vi "Config_interface.vi"() -> ()   [LabVIEW 2015]
uses:
  <vilib>/Utility/config.llb/NI_LVConfig.lvlib
  <vilib>/Utility/config.llb/Write Key (Double).vi
  <vilib>/Utility/config.llb/Write Key (String).vi
  <vilib>/Utility/config.llb/Write Key (U32).vi
  <vilib>/Utility/config.llb/Write Key (Boolean).vi
  <vilib>/LabVIEW Targets/FPGA/cRIO/shared/nicrio_ModuleControls/nicrio_cRIO-9233_DataRatesRing.ctl
panel:
  in  "Ruta en la que se quiere guardar el archivo parametros.cfg":path=path "Parametros.cfg"
  in  "Días entre TEST":i16(slide) scale=0.0..50.0
  in  "Horario":cluster{sgl, sgl, sgl}(slide)={61389.473, 53948.324, 46173.875} scale=0.0..86400.0 scale format="%<%H:%M>t"
  in  "Tab Control":T1(tab)=enum."Parámetros"
  in  "Frecuencia de muestreo (Hz)":dbl=50000.0
  in  "Escaneos de la FIFO por canal":u32=1000
  in  "Tiempo extra al detector de paso (s)":dbl=1.0
  in  "Filtro digital (ms)":u16=13
  in  "dt RMS":dbl=500.0
  in  "Data Rate":T2=2 items=["50.000 kS/s (NI 9233)"=2, "33.333 kS/s (NI 9233)"=3, "25.000 kS/s (NI 9233)"=34, "16.667 kS/s (NI 9233)"=35, "12.500 kS/s (NI 9233)"=36, "10.000 kS/s (NI 9233)"=37, "  8.333 kS/s (NI 9233)"=38, "  7.143 kS/s (NI 9233)"=39, "  6.250 kS/s (NI 9233)"=40, "  5.556 kS/s (NI 9233)"=41, "  5.000 kS/s (NI 9233)"=42, "  4.545 kS/s (NI 9233)"=43, "  4.167 kS/s (NI 9233)"=44, "  3.846 kS/s (NI 9233)"=45, "  3.571 kS/s (NI 9233)"=46, "  3.333 kS/s (NI 9233)"=47, "  3.125 kS/s (NI 9233)"=48, "  2.941 kS/s (NI 9233)"=49, "  2.778 kS/s (NI 9233)"=50, "  2.632 kS/s (NI 9233)"=51, "  2.500 kS/s (NI 9233)"=52, "  2.381 kS/s (NI 9233)"=53, "  2.273 kS/s (NI 9233)"=54, "  2.174 kS/s (NI 9233)"=55, "  2.083 kS/s (NI 9233)"=56, "  2.000 kS/s (NI 9233)"=57]
  in  "Puerto de conexión RFID":u16=2189
  in  "IP de RFID":string="192.168.100.2"
  in  "Hora de descarga":string="HH:MM"
  in  "Periodo descarga\n (Días)":u16=3
  in  "Descarga automática 2":bool
  in  "Hora de descarga":string="HH:MM"
  in  "Descarga automática":bool
  in  "Password FTP":string="crioftp"
  in  "Username FTP":string="crioftp"
  in  "Puerto FTP":u16=2121
  in  "IP del servidor FTP":string="80.39.98.109"
  in  "Puerto TCP/IP":u16=2122
  in  "IP del servidor FTP 2":string="80.39.98.109"
  in  "Username FTP 2":string="crioftp"
  in  "Password FTP 2":string="crioftp"
  in  "Puerto FTP 2":u16=2121
  in  "Periodo  de borrado de\narchivos (Días)":u16=5
  out "error out":errorcluster
  out "Horario TEST":string
  out "Horario inicio":string
  out "Horario final":string
  # "Funciona?"
  # "Inductivo"
  # "A4"
  # "A3"
  # "A1"
  # "A2"
  # "Inicio"
  # "Final"
  # "TEST"
  # "Dcha"
  # "Izda"
  # "Última detección de unidad"
  # "Error!!"
  # "Estado de la memoria"
  # "Parámetros de muestreo"
  # "Parámetros de adquisición"
  # "Parámetros de RFID"
  # "Cambio Fecha y Hora"
  # "Descarga de planos y TEST"
  # "NO"
  # "SI"
  # "Descarga archivos binarios de adquisición"
  # "NO"
  # "SI"
  # "Cargar datos de configuración"
  # "Errores!!"
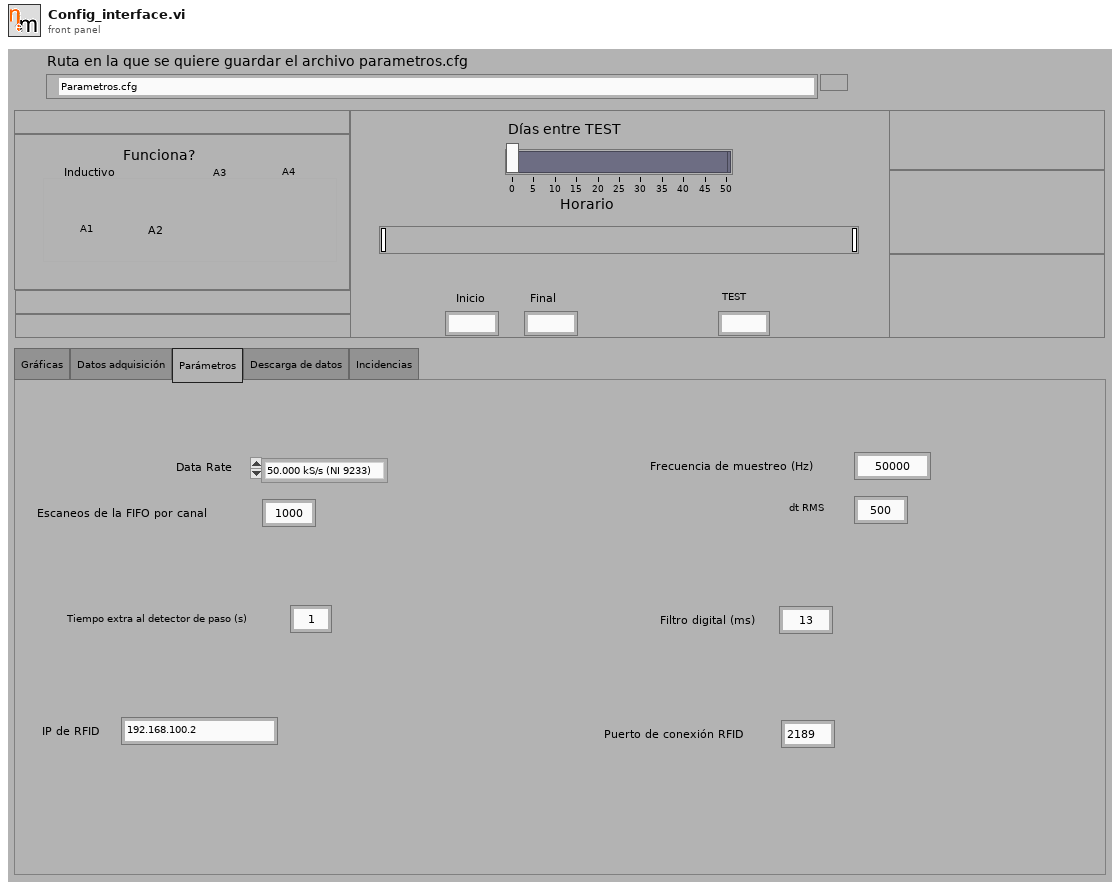
[diagram p1: front panel]
types:
  T1 = enum32{"Gráficas", "Datos adquisición", "Parámetros", "Descarga de datos", "Incidencias"}
  T2 = typedef "nicrio_cRIO-9233_DataRatesRing.ctl" = u8
  T3 = typedef "NI_LVConfig.lvlib/Config Data RefNum.ctl" = refnum<k1>
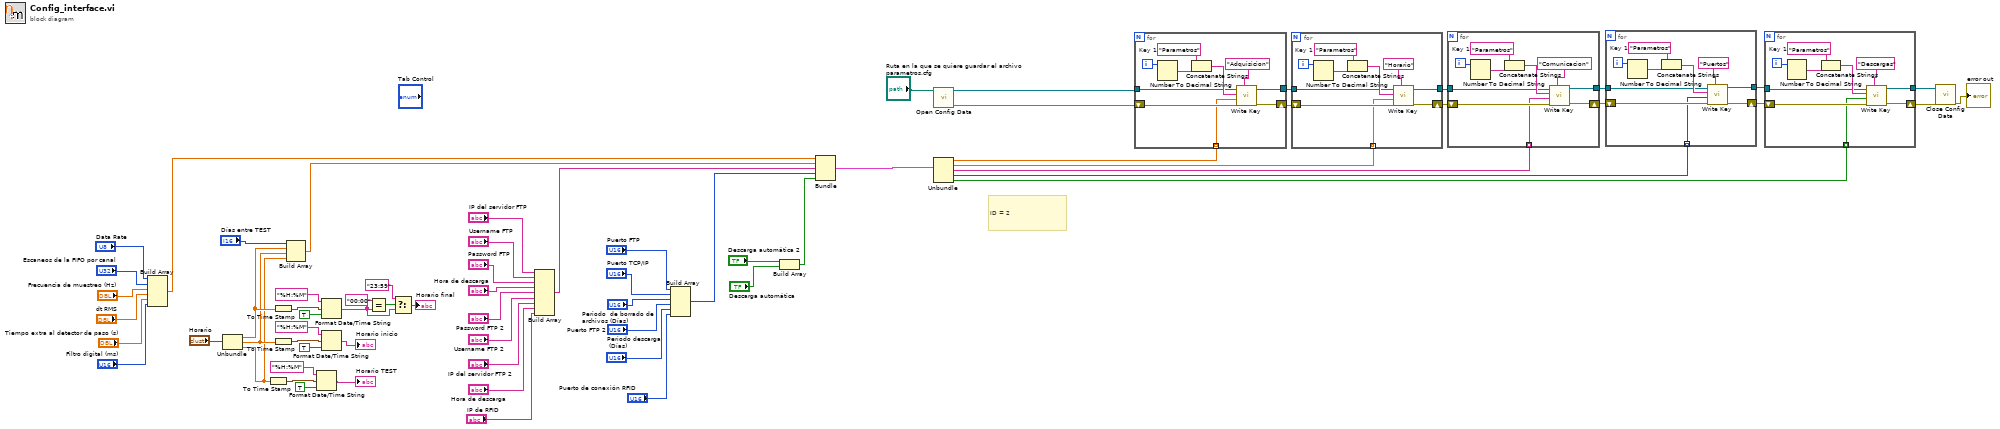
[diagram p0: block diagram]
diagram:
  # "ID = 2"
  n1 = Build Array("Data Rate", "Escaneos de la FIFO por canal", "Frecuencia de muestreo (Hz)", "dt RMS", "Tiempo extra al detector de paso (s)", "Filtro digital (ms)") -> (w28:dbl[])
  n2 = Unbundle("Horario") -> (w48:sgl, w46:sgl, w45:sgl)
  n3 = To Time Stamp(1:w45) -> (0:w60:timestamp)
  n4 = To Time Stamp(1:w48) -> (0:w67:timestamp)
  n5 = To Time Stamp(1:w46) -> (0:w64:timestamp)
  n6 = Build Array("Días entre TEST", w48, w46, w45) -> (w27:sgl[])
  n7 = Format Date/Time String(time format string (%c)="%H:%M", seconds (now)=w60, UTC format=TRUE) -> (date/time string=→"Horario TEST":string)
  n8 = Format Date/Time String(time format string (%c)="%H:%M", seconds (now)=w67, UTC format=TRUE) -> (date/time string=w56:string)
  n9 = Format Date/Time String(time format string (%c)="%H:%M", seconds (now)=w64, UTC format=TRUE) -> (date/time string=→"Horario inicio":string)
  n10 = Equal?(x="00:00" ("y"), y=w56) -> (x = y?=w58:bool)
  n11 = Select(t="23:59" ("y"), s=w58, f=w56) -> (s? t:f=→"Horario final":string)
  n12 = Build Array("IP del servidor FTP", "Username FTP", "Password FTP", "Hora de descarga", "Password FTP 2", "Username FTP 2", "IP del servidor FTP 2", "Hora de descarga", "IP de RFID") -> (w26:string[])
  n13 = Build Array("Puerto FTP", "Puerto TCP/IP", "Periodo  de borrado de\narchivos (Días)", "Puerto FTP 2", "Periodo descarga\n (Días)", "Puerto de conexión RFID") -> (w25:u16[])
  n14 = Build Array("Descarga automática 2", "Descarga automática") -> (w24:bool[])
  n15 = Bundle(w28, w27, w26, w25, w24) -> (w1:cluster{dbl[], sgl[], string[], u16[], bool[]})  [unwired: 1 in]
  n16 = Unbundle(w1) -> (w6:dbl[], w5:sgl[], w4:string[], w3:u16[], w2:bool[])
  n17 = call <vilib>:"Open Config Data.vi"("configuration file path"="Ruta en la que se quiere guardar el archivo parametros.cfg") -> ("error out"=w7:errorcluster, "refnum"=w8:T3)  [unwired: 2 in, 7 out]
  n18 = for {
    tunnel: w8 -> [w74]
    tunnel: w6 -> [w72] mode=indexing
    shift-right: [w71] -> w11
    shift-left: w7 -> [w73]
    tunnel: [w70] -> w10
    i -> [w78]
    w76 = "Parametros"  # Key 1
    n19 = Number To Decimal String(number=w78) -> (decimal integer string=w77:string)  [unwired: 1 in]
    n20 = Concatenate Strings(w76, w77) -> (w75:string)
    n21 = call-poly <vilib>:"Write Key.vi"("section"="Adquisicion", "error in (no error)"=w73, "value"=w72, "key"=w75, "refnum"=w74) -> ("error out"=w71:errorcluster, "refnum out"=w70:T3)  [unwired: 3 in, 2 out]
  }
  n22 = for {
    tunnel: w10 -> [w84]
    tunnel: w5 -> [w82] mode=indexing
    shift-right: [w81] -> w13
    shift-left: w11 -> [w83]
    tunnel: [w80] -> w12
    i -> [w88]
    w86 = "Parametros"  # Key 1
    n23 = Number To Decimal String(number=w88) -> (decimal integer string=w87:string)  [unwired: 1 in]
    n24 = Concatenate Strings(w86, w87) -> (w85:string)
    n25 = call-poly <vilib>:"Write Key.vi"("section"="Horario", "error in (no error)"=w83, "value"=w82, "key"=w85, "refnum"=w84) -> ("error out"=w81:errorcluster, "refnum out"=w80:T3)  [unwired: 3 in, 2 out]
  }
  n26 = for {
    tunnel: w12 -> [w94]
    tunnel: w4 -> [w90] mode=indexing
    shift-right: [w92] -> w15
    shift-left: w13 -> [w93]
    tunnel: [w91] -> w14
    i -> [w98]
    w96 = "Parametros"  # Key 1
    n27 = Number To Decimal String(number=w98) -> (decimal integer string=w97:string)  [unwired: 1 in]
    n28 = Concatenate Strings(w96, w97) -> (w95:string)
    n29 = call-poly <vilib>:"Write Key.vi"("section"="Comunicacion", "error in (no error)"=w93, "value"=w90, "key"=w95, "refnum"=w94) -> ("error out"=w92:errorcluster, "refnum out"=w91:T3)  [unwired: 1 in, 4 out]
  }
  n30 = for {
    tunnel: w14 -> [w104]
    tunnel: w3 -> [w100] mode=indexing
    shift-right: [w102] -> w17
    shift-left: w15 -> [w103]
    tunnel: [w101] -> w16
    i -> [w108]
    w106 = "Parametros"  # Key 1
    n31 = Number To Decimal String(number=w108) -> (decimal integer string=w107:string)  [unwired: 1 in]
    n32 = Concatenate Strings(w106, w107) -> (w105:string)
    n33 = call-poly <vilib>:"Write Key.vi"("section"="Puertos", "error in (no error)"=w103, "value"=w100, "key"=w105, "refnum"=w104) -> ("error out"=w102:errorcluster, "refnum out"=w101:T3)  [unwired: 5 out]
  }
  n34 = for {
    tunnel: w16 -> [w114]
    tunnel: w2 -> [w110] mode=indexing
    shift-right: [w112] -> w19
    shift-left: w17 -> [w113]
    tunnel: [w111] -> w18
    i -> [w118]
    w116 = "Parametros"  # Key 1
    n35 = Number To Decimal String(number=w118) -> (decimal integer string=w117:string)  [unwired: 1 in]
    n36 = Concatenate Strings(w116, w117) -> (w115:string)
    n37 = call-poly <vilib>:"Write Key.vi"("section"="Descargas", "error in (no error)"=w113, "value"=w110, "key"=w115, "refnum"=w114) -> ("error out"=w112:errorcluster, "refnum out"=w111:T3)  [unwired: 5 out]
  }
  n38 = call <vilib>:"Close Config Data.vi"("error in (no error)"=w19, "refnum"=w18) -> ("error out"=→"error out":errorcluster)  [unwired: 8 in, 1 out]
